vi "Configure Modulation (ASK).vi"(0 "VISA resource name":refnum<visa-resource-name>, 1 "Enable ASK Modulation (T: Enable)":bool=TRUE, 5 "Channel (1: Channel 1)":u16(ring)=1 items=["Channel 1"=1, "Channel 2"=2], 7 "ASK Modulation Source (0: Internal)":u16(ring) items=["Internal", "External"], 9 "Modulation Amplitude (1.00 Vpp)":dbl=1.0 format="%.2f", 11 "error in (no error)":errorcluster, 12 "Internal Rate (100.00 Hz)":dbl=100.0 format="%.2f") -> (4 "VISA resource name out":refnum<visa-resource-name>, 15 "error out":errorcluster)   [LabVIEW 2016, in "Tektronix AFG 1000 Series.lvlib"]
doc: "Configures and enables Amplitude-Shift Keying (ASK) modulation.\n\n<b>Note:</b>\nThis VI is not supported for AFG1022."
uses:
  Tektronix AFG 1000 Series.lvlib
panel:
  # "Internal ASK Settings"
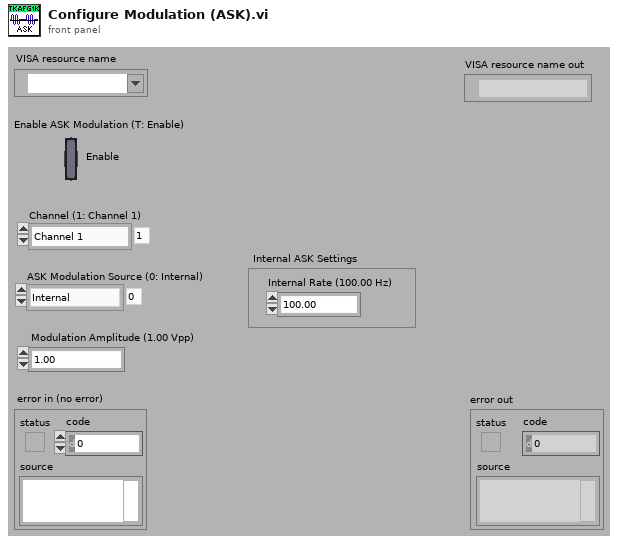
[diagram p1: front panel]
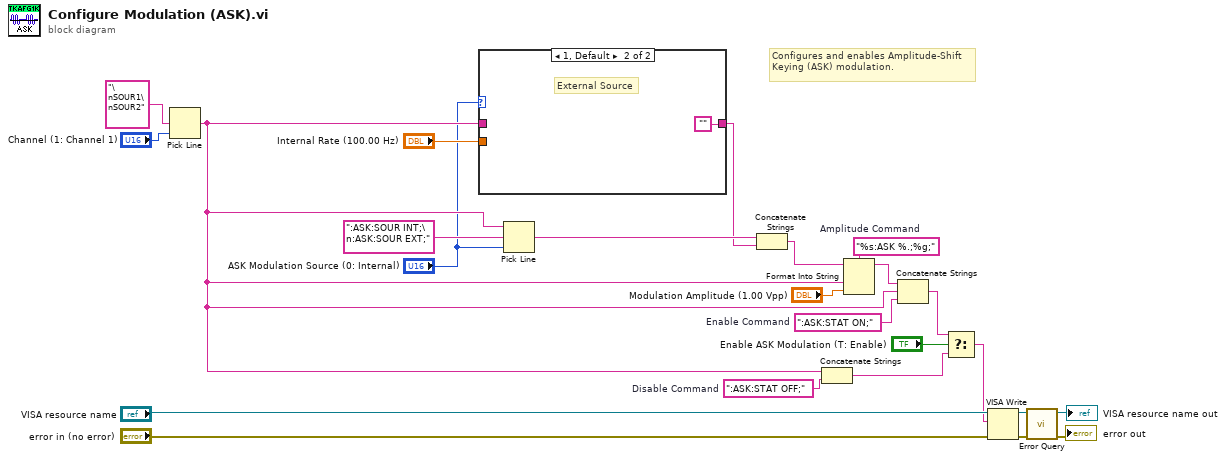
[diagram p0: block diagram]
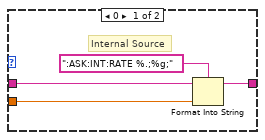
[diagram p2: hidden frame]
diagram:
  w17 = "%s:ASK %.;%g;"  # Amplitude Command
  w3 = ":ASK:STAT ON;"  # Enable Command
  w10 = ":ASK:STAT OFF;"  # Disable Command
  # "Configures and enables Amplitude-Shift Keying (ASK) modulation."
  n1 = Pick Line(multi-line string="\nSOUR1\nSOUR2" ("string (\"\")"), line index="Channel (1: Channel 1)") -> (output string=w2:string)  [unwired: 1 in]
  n2 = case shown="1, Default" "ASK Modulation Source (0: Internal)" {
    tunnel: [w27 ""] -> w7
    tunnel: w2 -> [w26 _]
    tunnel: "Internal Rate (100.00 Hz)" -> [w25 _]
    frame 0 {
      # "Internal Source"
      n3 = Format Into String(format string=":ASK:INT:RATE %.;%g;" ("initial string"), initial string=w26, w25) -> (resulting string=w27:string)  [unwired: 1 in, 1 out]
    }
    frame 1, Default {
      # "External Source"
    }
  }
  n4 = Pick Line(string ("")=w2, multi-line string=":ASK:SOUR INT;\n:ASK:SOUR EXT;" ("string (\"\")"), line index="ASK Modulation Source (0: Internal)") -> (output string=w8:string)
  n5 = Concatenate Strings(w8, w7) -> (w6:string)
  n6 = Concatenate Strings(w2, w10) -> (w9:string)
  n7 = Format Into String(format string=w17, initial string=w6, w2, "Modulation Amplitude (1.00 Vpp)") -> (resulting string=w18:string)  [unwired: 1 in, 1 out]
  n8 = Concatenate Strings(w18, w2, w3) -> (w11:string)
  n9 = Select(t=w11, s="Enable ASK Modulation (T: Enable)", f=w9) -> (s? t:f=w12:string)
  n10 = VISA Write(VISA resource name="VISA resource name", write buffer=w12, error in (no error)="error in (no error)") -> (VISA resource name out=w23:refnum<visa-resource-name>, error out=w22:errorcluster)  [unwired: 1 out]
  n11 = call "Error Query.vi"("error in (no error)"=w22, "VISA resource name"=w23) -> ("error out"=→"error out":errorcluster, "VISA resource name out"=→"VISA resource name out":refnum<visa-resource-name>)  [unwired: 6 in, 2 out]
